vi "Write state.vi"(8 "error in (no error)":errorcluster, 10 "guideAutoclearStateTypes":T1, 11 "GuideAutoclearState in":refnum<class "GuideAutoclearState.lvclass">) -> (0 "error out":errorcluster, 3 "GuideAutoclearState out":refnum<class "GuideAutoclearState.lvclass">)   [LabVIEW 2022 SP3, in "TCSDataDefinitions.lvlib" / "TCSCommand.lvlib" / "GuiderCommands.lvlib" / "GuideAutoclearState.lvclass"]
uses:
  GuideAutoclearState.lvclass
  Enumerations/GuideAutoclearStateTypes.ctl
  GuideAutoclearState.lvclass/GuideAutoclearState.ctl
  TCSCommand.lvlib
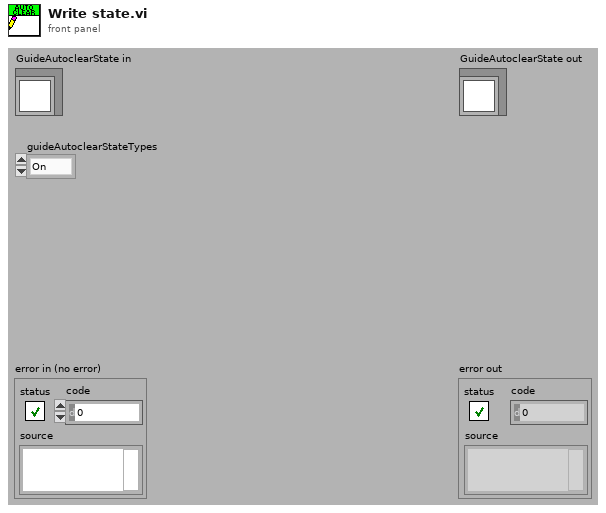
[diagram p1: front panel]
types:
  T1 = typedef "TCSDataDefinitions.lvlib/TCSCommand.lvlib/GuideAutoclearStateTypes.ctl" = enum16{"On", "Off"}
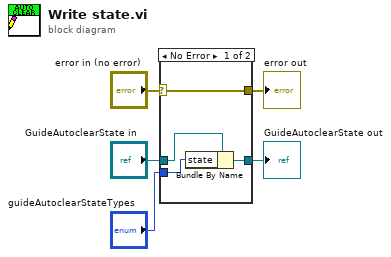
[diagram p0: block diagram]
diagram:
  n1 = case shown="No Error" "error in (no error)" {
    selector: "error in (no error)" -> [w9 w10]
    tunnel: [w9 w10] -> w4
    tunnel: [w7 w11] -> w2
    tunnel: "GuideAutoclearState in" -> [w8 w11]
    tunnel: "guideAutoclearStateTypes" -> [w6 _]
    frame No Error {
      n2 = Bundle By Name(cluster=w8, "state"=w6) -> (w7:refnum<class "GuideAutoclearState.lvclass">)
    }
    frame Error {
    }
  }
  "error out" <- w4
  "GuideAutoclearState out" <- w2
